vi "onInterruptProcessTriggers.vi"(8 "error in (no error)":errorcluster, 10 "model in":refnum<class "IModel.lvclass">, 11 "DisabledState in":refnum<class "DisabledState.lvclass">) -> (0 "error out":errorcluster, 2 "model out":refnum<class "IModel.lvclass">, 3 "DisabledState out":refnum<class "DisabledState.lvclass">)   [LabVIEW 2016, in "States.lvlib" / "DisabledState.lvclass"]
uses:
  DisabledState.lvclass
  IModel/IModel.lvclass
  ts_sallv_sedspectrometer/DataTypes/logevent_SummaryState.ctl
  ts_sallv_sedspectrometer/DataTypes/logevent_DetailedState.ctl
  ts_sallv_sedspectrometer/SALLV_sedSpectrometer.lvlib
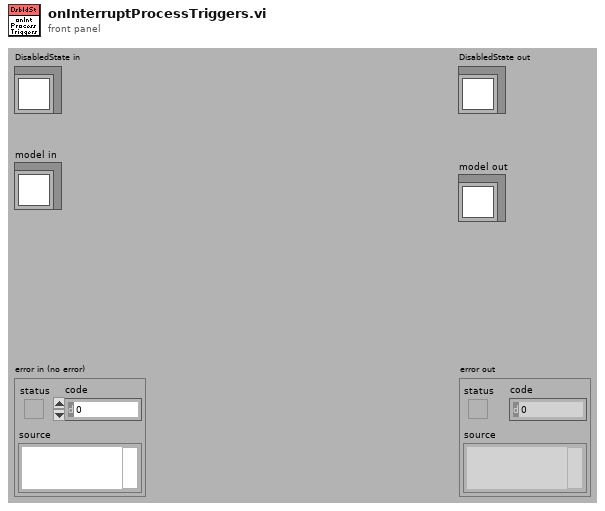
[diagram p1: front panel]
types:
  T1 = typedef "SALLV_sedSpectrometer.lvlib/logevent_DetailedState.ctl" = cluster{"detailedState":enum16{"", "DisabledState", "EnabledState", "FaultState", "OfflineState", "StandbyState"}, "priority":i32}
  T2 = typedef "SALLV_sedSpectrometer.lvlib/logevent_SummaryState.ctl" = cluster{"summaryState":enum16{"", "DisabledState", "EnabledState", "FaultState", "OfflineState", "StandbyState"}, "priority":i32}
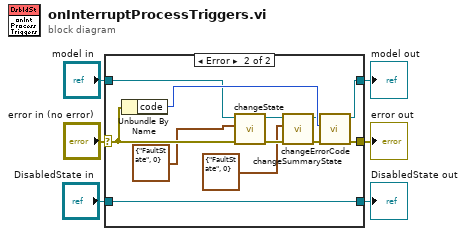
[diagram p0: block diagram]
diagram:
  n1 = case shown="Error" "error in (no error)" {
    selector: "error in (no error)" -> [w9 w20]
    tunnel: [w9 w17] -> w5
    tunnel: [w8 w12] -> w4
    tunnel: "model in" -> [w8 w15]
    tunnel: [w7 w16] -> w2
    tunnel: "DisabledState in" -> [w7 w16]
    frame No Error {
    }
    frame Error {
      n2 = Unbundle By Name(w20) -> ("code"=w21:i32)
      n3 = call-dynamic "changeState.vi"("error in (no error)"=w20, "DetailedState"=T1 {"detailedState"=enum."FaultState", "priority"=0} ("logevent_DetailedState"), "IModel in"=w15) -> ("error out"=w19:errorcluster, "IModel out"=w14:refnum<class "IModel.lvclass">)  [unwired: 7 in]
      n4 = call-dynamic "changeSummaryState.vi"("error in (no error)"=w19, "logevent_SummaryState"=T2 {"summaryState"=enum."FaultState", "priority"=0}, "IModel in"=w14) -> ("error out"=w18:errorcluster, "IModel out"=w13:refnum<class "IModel.lvclass">)  [unwired: 7 in]
      n5 = call-dynamic "changeErrorCode.vi"("error in (no error)"=w18, "error.code"=w21, "IModel in"=w13) -> ("error out"=w17:errorcluster, "IModel out"=w12:refnum<class "IModel.lvclass">)  [unwired: 7 in]
    }
  }
  "error out" <- w5
  "DisabledState out" <- w2
  "model out" <- w4
